vi "Hold.vi"(8 "error in (no error)":errorcluster, 11 "PS Control Actor in":refnum<class "PS Control Actor.lvclass">) -> (0 "error out":errorcluster, 3 "PS Control Actor out":refnum<class "PS Control Actor.lvclass">)   [LabVIEW 2025, in "PS Control Actor.lvlib" / "PS Control Actor.lvclass"]
doc: "Author: Scott Hannahs <sth@magnet.fsu.edu>\n\nThis software is licensed for use under the “MIT License\"\nCopyright (c) 2025 Scott Hannahs, sth@sth@magnet.sthnet.net\n\nPermission is hereby granted, free of charge, to any person obtaining a copy of this software and associated documentation files (the \"Software\"), to deal in the Software without restriction, including without limitation the rights to use, copy, modify, merge, publish, distribute, sublicense, and/or sell copies of the Software, and to permit persons to whom the Software is furnished to do so, subject to the following conditions: The above copyright notice and this permission notice shall be included in all copies or substantial portions of the Software.\n\nTHE SOFTWARE IS PROVIDED \"AS IS\", WITHOUT WARRANTY OF ANY KIND, EXPRESS OR IMPLIED, INCLUDING BUT NOT LIMITED TO THE WARRANTIES OF MERCHANTABILITY, FITNESS FOR A PARTICULAR PURPOSE AND NONINFRINGEMENT. IN NO EVENT SHALL THE AUTHORS OR COPYRIGHT HOLDERS BE LIABLE FOR ANY CLAIM, DAMAGES OR OTHER LIABILITY, WHETHER IN AN ACTION OF CONTRACT, TORT OR OTHERWISE, ARISING FROM, OUT OF OR IN CONNECTION WITH THE SOFTWARE OR THE USE OR OTHER DEALINGS IN THE SOFTWARE."
uses:
  PS Control Actor.lvclass
  PS Control Actor.lvclass/PS Control Actor.ctl
  PS Driver/PS Driver.lvclass
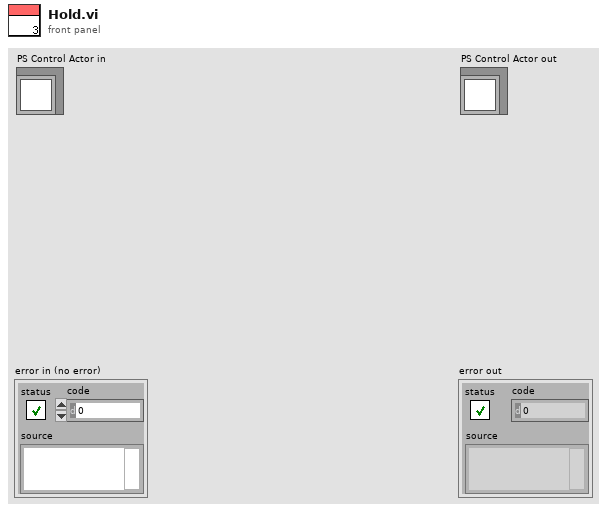
[diagram p1: front panel]
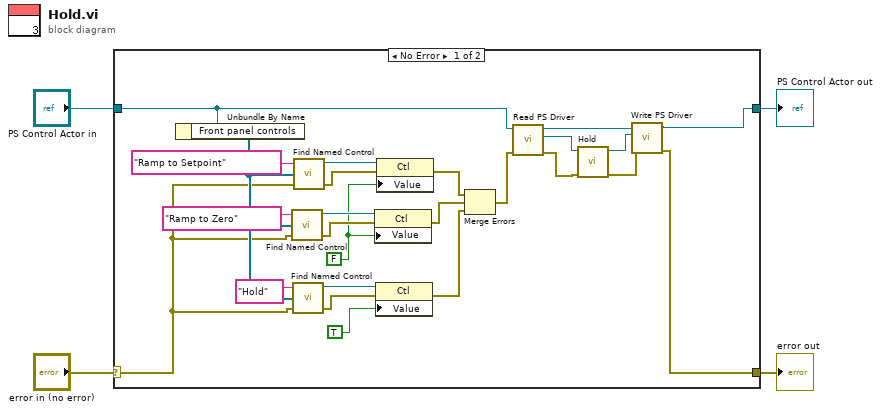
[diagram p0: block diagram]
diagram:
  n1 = case shown="No Error" "error in (no error)" {
    selector: "error in (no error)" -> [w16 w31]
    tunnel: [w10 w31] -> w3
    tunnel: [w7 w30] -> w1
    tunnel: "PS Control Actor in" -> [w9 w30]
    frame No Error {
      w21 = FALSE
      n2 = Unbundle By Name(w9) -> ("Front panel controls"=w17:refnum<vi>[])
      n3 = call "Find Named Control.vi"("error in"=w16, "All Controls"=w17, "Control Name"="Ramp to Zero") -> ("error out"=w25:errorcluster, "Ctl Refnum"=w26:refnum<vi>)  [unwired: 1 out]
      n4 = call "Find Named Control.vi"("error in"=w16, "All Controls"=w17, "Control Name"="Hold") -> ("error out"=w19:errorcluster, "Ctl Refnum"=w20:refnum<vi>)  [unwired: 1 out]
      n5 = call "Find Named Control.vi"("error in"=w16, "All Controls"=w17, "Control Name"="Ramp to Setpoint") -> ("error out"=w28:errorcluster, "Ctl Refnum"=w29:refnum<vi>)  [unwired: 1 out]
      n6 = property class="Ctl"(reference=w26, error in=w25, "Value"=w21) -> (error out=w22:errorcluster)  [unwired: 1 out]
      n7 = property class="Ctl"(reference=w20, error in=w19, "Value"=TRUE) -> (error out=w14:errorcluster)  [unwired: 1 out]
      n8 = property class="Ctl"(reference=w29, error in=w28, "Value"=w21) -> (error out=w23:errorcluster)  [unwired: 1 out]
      n9 = Merge Errors(w23, w22, w14) -> (w13:errorcluster)
      n10 = call-dynamic "Read PS Driver.vi"("error in (no error)"=w13, "PS Control Actor in"=w9) -> ("error out"=w12:errorcluster, "PS Driver.lvlib:PS Driver.lvclass"=w6:refnum<class "PS Driver.lvclass">, "PS Control Actor out"=w8:refnum<class "PS Control Actor.lvclass">)  [unwired: 7 in]
      n11 = call-dynamic "Hold.vi"("error in (no error)"=w12, "PS Driver.lvlib:PS Driver.lvclass in"=w6) -> ("error out"=w11:errorcluster, "PS Driver.lvlib:PS Driver.lvclass out"=w5:refnum<class "PS Driver.lvclass">)  [unwired: 8 in]
      n12 = call-dynamic "Write PS Driver.vi"("error in (no error)"=w11, "PS Driver.lvlib:PS Driver.lvclass"=w5, "PS Control Actor in"=w8) -> ("error out"=w10:errorcluster, "PS Control Actor out"=w7:refnum<class "PS Control Actor.lvclass">)  [unwired: 7 in]
    }
    frame Error {
    }
  }
  "error out" <- w3
  "PS Control Actor out" <- w1
